vi "MovPlayer_v0.vi"() -> ()   [LabVIEW 2016]
uses:
  Global_InitEndSync.vi
  <vilib>/vision/NI_Vision_Development_Module.lvlib
panel:
  in  "No. of repeat":dbl=inf
  in  "Play Button":bool
  in  "Manual Stop Button":bool
  in  "Disp":bool[](array[boolean])=[FALSE, FALSE, FALSE, FALSE, FALSE, FALSE]
  in  "Project Path":path=path "C:/Users/FVMPE/Documents/LabVIEW_programs/3mBM/kit/v3/mov"
  out "State":string
  in  "error in":errorcluster
  # "#1"
  # "#2"
  # "#3"
  # "#4"
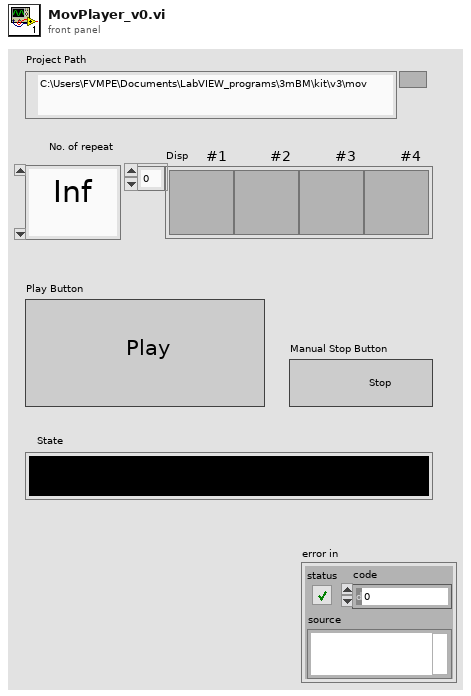
[diagram p1: front panel]
types:
  T1 = typedef "IMAQ AVI2 Refnum.ctl" = refnum<k20>
  T2 = cluster{"Width":u32, "Height":u32, "Frames Per Second":u32, "Codec":string, "Has Data":bool}
  T3 = typedef "Image Type" = u32
  T4 = typedef "IMAQ Image.ctl" = refnum<image>
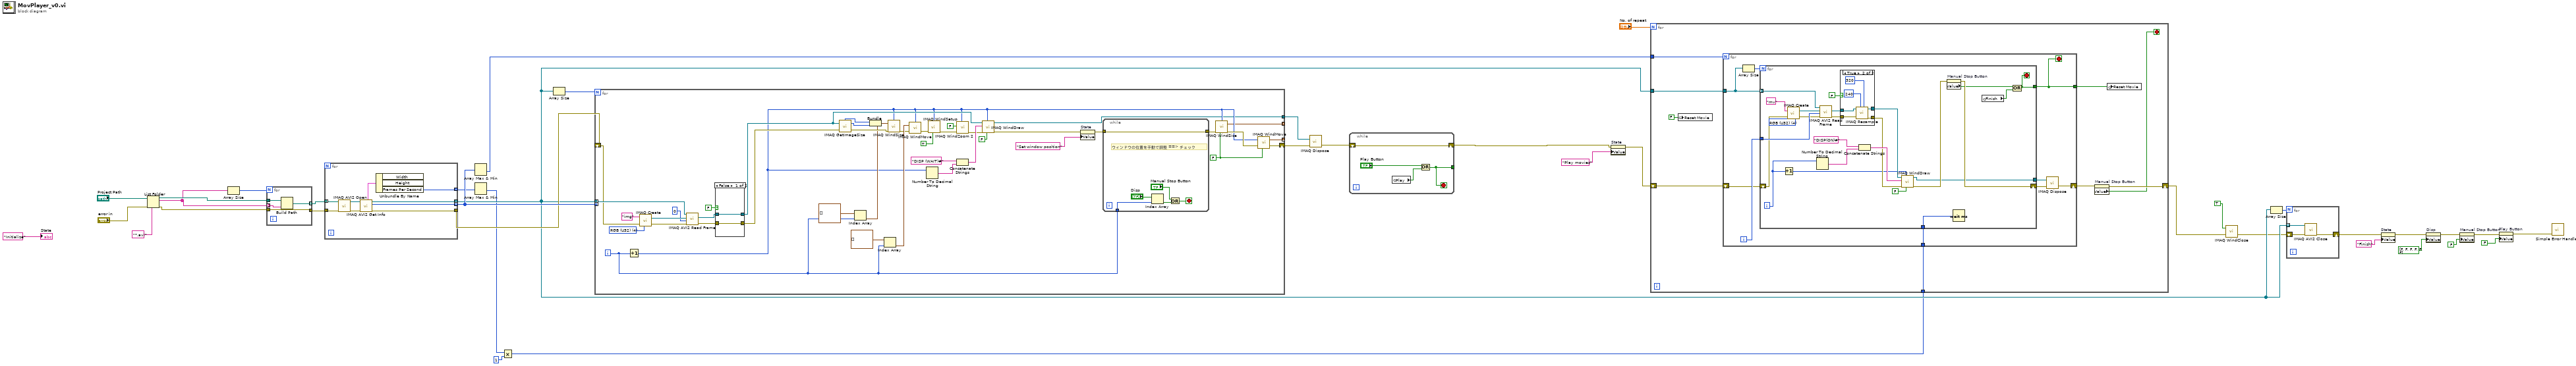
[diagram p0: block diagram]
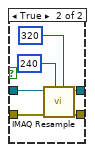
[diagram p3: hidden frame]
diagram:
  n1 = List Folder(path="Project Path", pattern="*.avi", error in="error in") -> (path out=w34:path, filenames=w33:string[], error out=w37:errorcluster)  [unwired: 1 in, 1 out]
  n2 = Array Size(array=w33) -> (size(s)=w32:i32)
  n3 = for {
    N: w32 -> [_]
    tunnel: w37 -> [w41]
    tunnel: [w40] -> w31 mode=indexing
    tunnel: [w41] -> w30
    tunnel: w34 -> [w43]
    tunnel: w33 -> [w42] mode=indexing
    n4 = Build Path(base path=w43, name or relative path=w42) -> (appended path=w40:path)
  }
  n5 = for {
    tunnel: w31 -> [w52] mode=indexing
    tunnel: w30 -> [w51]
    tunnel: [w48] -> w21 mode=indexing
    tunnel: [w47] -> w26
    tunnel: [w46] -> w27 mode=indexing
    tunnel: [w44] -> w19 mode=indexing
    n6 = call "IMAQ AVI2 Open"("error in (no error)"=w51, "AVI File Path"=w52) -> ("error out"=w49:errorcluster, "AVI Refnum"=w50:T1)  [unwired: 8 in]
    n7 = call "IMAQ AVI2 Get Info"("error in (no error)"=w49, "AVI Refnum"=w50) -> ("error out"=w47:errorcluster, "Number of Frames"=w46:u32, "AVI Refnum (duplicate)"=w48:T1, "Frame Data"=w45:T2)  [unwired: 5 in, 1 out]
    n8 = Unbundle By Name(w45) -> ("Frames Per Second"=w44:u32)  [unwired: 2 out]
  }
  n9 = Array Max & Min(array=w19) -> (min value=w18:u32)  [unwired: 3 out]
  n10 = Array Max & Min(array=w27) -> (min value=w28:u32)  [unwired: 3 out]
  n11 = Multiply(x=w18, y=1) -> (x*y=w5:u32)
  n12 = Array Size(array=w21) -> (size(s)=w29:i32)
  n13 = for {
    N: w29 -> [_]
    tunnel: w21 -> [w89] mode=indexing
    tunnel: w27 -> [_] mode=indexing
    shift-right: [w66] -> w3
    shift-left: w26 -> [w62]
    tunnel: [w61] -> _ mode=indexing
    tunnel: [w60] -> _ mode=indexing
    tunnel: [w53] -> w1
    i -> [w71]
    w55 = T3 4 items=["Grayscale (U8)", "Grayscale (I16)", "Grayscale (SGL)", "Complex (CSG)", "RGB (U32)", "HSL (U32)", "RGB (U64)", "Grayscale (U16)"] ("Image Type")
    w82 = FALSE
    n14 = Increment(x=w71) -> (x+1=w63:i32)
    n15 = call "IMAQ Create"("Image Name"="img", "Image Type"=w55, "error in (no error)"=w62) -> ("New Image"=w93:T4, "error out"=w92:errorcluster)  [unwired: 2 in]
    n16 = call "IMAQ AVI2 Read Frame"("error in (no error)"=w92, "Frame Number"=0, "Image"=w93, "AVI Refnum"=w89) -> ("error out"=w90:errorcluster, "Image Out"=w91:T4)  [unwired: 5 in, 1 out]
    n17 = case shown="False" FALSE {
      tunnel: w91 -> [w96 w102]
      tunnel: w90 -> [w95 w101]
      tunnel: [w96 w98] -> w68
      tunnel: [w95 w97] -> w67
      frame False {
      }
      frame True {
        n18 = call "IMAQ Resample"("X Resolution"=320, "Y Resolution"=240, "error in (no error)"=w101, "Image Src"=w102) -> ("error out"=w97:errorcluster, "Image Dst Out"=w98:T4)  [unwired: 6 in]
      }
    }
    n19 = call "IMAQ GetImageSize"("Image"=w68, "error in (no error)"=w67) -> ("Y Resolution"=w81:i32, "X Resolution"=w80:i32, "error out"=w76:errorcluster)  [unwired: 2 in]
    n20 = Index Array(array=cluster{"Width":i32, "Height":i32}[] [], index=w71) -> (element=w65:cluster{"Width":i32, "Height":i32})
    n21 = Bundle(cluster=w65, "Width"=w80, "Height"=w81) -> (w64:cluster{"Width":i32, "Height":i32})
    n22 = Index Array(array=cluster{"Width":i32, "Height":i32}[] [], index=w71) -> (element=w85:cluster{"Width":i32, "Height":i32})
    n23 = call "IMAQ WindSize"("error in (no error)"=w76, "Width & Height"=w64, "Window Number"=w63) -> ("error out"=w77:errorcluster)  [unwired: 3 in, 2 out]
    n24 = call "IMAQ WindMove"("Window Number (0...15)"=w63, "Coordinates (screen)"=w85, "error in (no error)"=w77) -> ("error out"=w79:errorcluster)  [unwired: 2 in, 1 out]
    n25 = Number To Decimal String(number=w63) -> (decimal integer string=w87:string)  [unwired: 1 in]
    n26 = call "IMAQ WindSetup"("Window is floating? (No)"=TRUE, "Window Number (0...15)"=w63, "error in (no error)"=w79) -> ("error out"=w74:errorcluster)  [unwired: 8 in]
    n27 = call "IMAQ WindZoom 2"("Window Number (0...15)"=w63, "error in (no error)"=w74, "Zoom to Fit? (False)"=FALSE) -> ("error out"=w75:errorcluster)  [unwired: 5 in, 3 out]
    n28 = Concatenate Strings("DISP (WAIT)#", w87) -> (w86:string)
    n29 = call "IMAQ WindDraw"("Resize to Image Size? (Y)"=FALSE, "Window Number (0...15)"=w63, "error in (no error)"=w75, "Title"=w86, "Image"=w68) -> ("error out"=w54:errorcluster, "Image Out (duplicate)"=w53:T4)  [unwired: 5 in]
    n30 = property on="State" class="Str"(error in=w54, "Value"="Set window position") -> (error out=w58:errorcluster)  [unwired: 1 in, 1 out]
    n31 = while {
      tunnel: w71 -> [w108]
      tunnel: [w103] -> w84
      tunnel: w58 -> [w103]
      stop <- w106 stop-if-true
      # "ウィンドウの位置を手動で調整 ==> チェック"
      n32 = Index Array(array="Disp", index=w108) -> (element=w107:bool)
      n33 = Or(x="Manual Stop Button", y=w107) -> (x .or. y?=w106:bool)
    }
    n34 = call "IMAQ WindSize"("error in (no error)"=w84, "Get/Set Status? (Set)"=w82, "Window Number"=w63) -> ("error out"=w83:errorcluster, "Width & Height out"=w61:cluster{"Width":i32, "Height":i32})  [unwired: 3 in, 1 out]
    n35 = call "IMAQ WindMove"("Window Number (0...15)"=w63, "Get/Set Status? (Set)"=w82, "error in (no error)"=w83) -> ("Coordinates (screen)"=w60:cluster{"X Position":i32, "Y Position":i32}, "error out"=w66:errorcluster)  [unwired: 2 in]
  }
  n36 = call "IMAQ Dispose"("Image"=w1, "error in (no error)"=w3) -> ("error out"=w2:errorcluster)  [unwired: 4 in]
  n37 = while {
    shift-right: [w111] -> w25
    shift-left: w2 -> [w111]
    tunnel: [w109] -> _
    stop <- w109 stop-if-true
    n38 = global read "Global_InitEndSync.vi" "Play"() -> (w110:bool)
    n39 = Or(x="Play Button", y=w110) -> (x .or. y?=w109:bool)
  }
  n40 = property on="State" class="Str"(error in=w25, "Value"="Play movies") -> (error out=w16:errorcluster)  [unwired: 1 in, 1 out]
  n41 = for {
    N: "No. of repeat" -> [_]
    tunnel: w28 -> [w121]
    tunnel: w21 -> [w120]
    tunnel: w5 -> [w119]
    shift-right: [w116] -> w23
    shift-left: w16 -> [w118]
    stop <- w114 stop-if-true
    n42 = global write "Global_InitEndSync.vi" "Reset Movie"(FALSE) -> ()
    n43 = for {
      N: w121 -> [_]
      tunnel: w120 -> [w125]
      shift-right: [w123] -> w117
      shift-left: w118 -> [w128]
      tunnel: w119 -> [w127]
      tunnel: [w122] -> w115
      i -> [w130]
      stop <- w122 stop-if-true
      n44 = Array Size(array=w125) -> (size(s)=w126:i32)
      n45 = for {
        N: w126 -> [_]
        tunnel: w130 -> [w153]
        tunnel: w125 -> [w152] mode=indexing
        shift-right: [w137] -> w129
        shift-left: w128 -> [w140]
        tunnel: w127 -> [w139]
        tunnel: [w134] -> w124
        tunnel: [w132] -> w122
        i -> [w146]
        stop <- w132 stop-if-true
        w136 = T3 4 items=["Grayscale (U8)", "Grayscale (I16)", "Grayscale (SGL)", "Complex (CSG)", "RGB (U32)", "HSL (U32)", "RGB (U64)", "Grayscale (U16)"] ("Image Type")
        n46 = Increment(x=w146) -> (x+1=w144:i32)
        n47 = call "IMAQ Create"("Image Name"="mv", "Image Type"=w136, "error in (no error)"=w140) -> ("New Image"=w142:T4, "error out"=w141:errorcluster)  [unwired: 2 in]
        n48 = Number To Decimal String(number=w146) -> (decimal integer string=w151:string)  [unwired: 1 in]
        n49 = call "IMAQ AVI2 Read Frame"("error in (no error)"=w141, "Frame Number"=w153, "Image"=w142, "AVI Refnum"=w152) -> ("error out"=w154:errorcluster, "Image Out"=w155:T4)  [unwired: 5 in, 1 out]
        n50 = case shown="True" FALSE {
          tunnel: w155 -> [w157 w163]
          tunnel: w154 -> [w156 w162]
          tunnel: [w156 w159] -> w148
          tunnel: [w157 w158] -> w147
          frame False {
          }
          frame True {
            n51 = call "IMAQ Resample"("X Resolution"=320, "Y Resolution"=240, "error in (no error)"=w162, "Image Src"=w163) -> ("error out"=w159:errorcluster, "Image Dst Out"=w158:T4)  [unwired: 6 in]
          }
        }
        n52 = Concatenate Strings("DISP(ON)#", w151) -> (w149:string)
        n53 = call "IMAQ WindDraw"("Resize to Image Size? (Y)"=FALSE, "Window Number (0...15)"=w144, "error in (no error)"=w148, "Title"=w149, "Image"=w147) -> ("error out"=w138:errorcluster, "Image Out (duplicate)"=w134:T4)  [unwired: 5 in]
        n54 = property on="Manual Stop Button" class="Bool (strict)"(error in=w138) -> (error out=w137:errorcluster, "Value"=w133:bool)  [unwired: 1 in, 1 out]
        n55 = Wait (ms)(milliseconds to wait=w139) -> ()  [unwired: 1 out]
        n56 = global read "Global_InitEndSync.vi" "Finish"() -> (w131:bool)
        n57 = Compound Arithmetic op=OR(w133, w131) -> (w132:bool)
      }
      n58 = call "IMAQ Dispose"("Image"=w124, "error in (no error)"=w129) -> ("error out"=w123:errorcluster)  [unwired: 4 in]
    }
    n59 = property on="Manual Stop Button" class="Bool (strict)"(error in=w117) -> (error out=w116:errorcluster, "Value"=w114:bool)  [unwired: 1 in, 1 out]
    n60 = global write "Global_InitEndSync.vi" "Reset Movie"(w115) -> ()
  }
  n61 = call "IMAQ WindClose"("Close All Windows (False)"=TRUE, "error in (no error)"=w23) -> ("error out"=w20:errorcluster)  [unwired: 4 in]
  n62 = Array Size(array=w21) -> (size(s)=w22:i32)
  n63 = for {
    N: w22 -> [_]
    tunnel: w21 -> [w166] mode=indexing
    shift-right: [w165] -> w13
    shift-left: w20 -> [w164]
    n64 = call "IMAQ AVI2 Close"("error in (no error)"=w164, "AVI Refnum"=w166) -> ("error out"=w165:errorcluster)  [unwired: 9 in]
  }
  n65 = property on="State" class="Str"(error in=w13, "Value"="Finish") -> (error out=w12:errorcluster)  [unwired: 1 in, 1 out]
  n66 = property on="Disp" class="Arr (strict)"(error in=w12, "Value"=bool[] [FALSE, FALSE, FALSE, FALSE, FALSE, FALSE] ("Disp")) -> (error out=w10:errorcluster)  [unwired: 1 in, 1 out]
  n67 = property on="Manual Stop Button" class="Bool (strict)"(error in=w10, "Value"=FALSE) -> (error out=w9:errorcluster)  [unwired: 1 in, 1 out]
  n68 = property on="Play Button" class="Bool (strict)"(error in=w9, "Value"=FALSE ("Play Button")) -> (error out=w8:errorcluster)  [unwired: 1 in, 1 out]
  n69 = call <vilib>:"Simple Error Handler.vi"("error in (no error)"=w8) -> ()  [unwired: 4 in, 5 out]
  "State" <- "Initialize"
